vi "CLSUIP_SetNmdUnbundlerElement.vi"(8 "error in (no error)":errorcluster, 10 "Element Names":string[](array[string]), 11 "NmdUnbundler Ref":refnum<vi>) -> (0 "error out":errorcluster, 3 "NmdUnbundler Ref out":refnum<vi>)   [LabVIEW 2019, in "BlueBranch_CLSUIP.lvlib"]
uses:
  BlueBranch_CLSUIP.lvlib
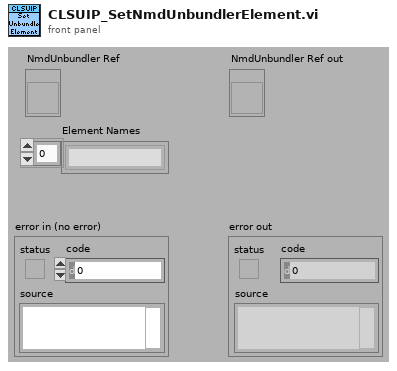
[diagram p1: front panel]
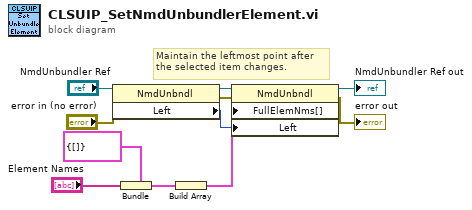
[diagram p0: block diagram]
diagram:
  # "Maintain the leftmost point after\nthe selected item changes."
  n1 = property class="NmdUnbndl"(reference="NmdUnbundler Ref", error in="error in (no error)") -> (reference out=w9:refnum<vi>, error out=w1:errorcluster, "Left"=w6:i32)
  n2 = Bundle(cluster=cluster{string[]} {[]}, "Element Names") -> (w3:cluster{string[]})
  n3 = Build Array(w3) -> (w2:cluster{string[]}[])
  n4 = property class="NmdUnbndl"(reference=w9, error in=w1, "FullElemNms[]"=w2, "Left"=w6) -> (reference out=→"NmdUnbundler Ref out":refnum<vi>, error out=→"error out":errorcluster)
